vi "Execute New VI From Template.vi"(6 "Mouse Position":T2, 8 "User VI Ref":refnum<vi>, 9 "Menu Item Tag Suffix":string, 10 "Remaining Items":refnum<vi>[](array[refnum]), 11 "Affected Items":cluster{"Any Refnums":refnum<vi>[]}) -> (0 "Fail transaction?":bool)   [LabVIEW 2022 SP3]
doc: "This is the main VI of the \"New VI From Template\" shortcut menu plugin.\n\nNotes from shortcut menu template VI:\n1. This VI has no need for a Close Reference call because GObject refnums do not hold the VI in memory. The User VI Ref will be closed by the caller.\n2. You may enable debugging on this VI to help develop your code. Debugging only has to be disabled on the builder VI, not the execute VI.\n\nPetru Tarabuta, Robusto Systems, September 2022"
uses:
  <vilib>/Utility/miscctls.llb/LVPositionTypeDef.ctl
  Owner Status (enum).ctl
  GUI Objects (cluster).ctl
  Testing Flag (enum).ctl
  Testing Flag (library variable).vi
  <resource>/Framework/Providers/VILibrary/LIBUIP_item_type.ctl
panel:
  out "Application Name":string
  out "VI Of Top-Most Block Diagram":string
  out "This Application Reference":u32
  out "Application Name":string
  out "VI Of Top-Most Block Diagram":string
  out "This Application Reference":u32
  in  "SCL":i32(listbox) caption="Template VIs and CTLs"
  in  "Apply Owner Icon Template?":bool
  out "Error Out":errorcluster
  out "Owner Filename (including extension)":string
  out "User VI Owner Status":T1
  out "Owner Path":path
  out "Iteration":i32
  out "Tab":enum32{"SomeTemplatesFound", "NoTemplatesFound"}(tab)
  in  "Insert into Virtual Folder?":bool
  in  "Create Button":bool
  in  "Destination Location":path caption="Destination Folder"
  in  "Project ComboBox":string(combo) caption="Project"
  in  "New Filename":string
  in  "VI Description":string
  in  "Add To Project?":bool
  in  "Add To Owner?":bool caption="Add to Class 1.lvclass?"
  in  "Open Front Panel?":bool caption="Open Front Panel When Created?"
  out "Virtual Folder Path":string
  out "NoTemplatesFound Message":string
  in  "Front Panel Sizing Tool":bool
  # "Execute VI"
  # "The tool's Application Instance"
  # "The User VI's Application Instance"
  # "The section below is not user-facing. For developer use only."
  # "All controls on this panel except \"Affected Items\" have been locked to prevent accidental edits. Changing the control names or types, other than the elements of the \"Affected Items\" cluster will make the VI unusable as a menu plugin.\n\nSee Context Help for each control for details about its use."
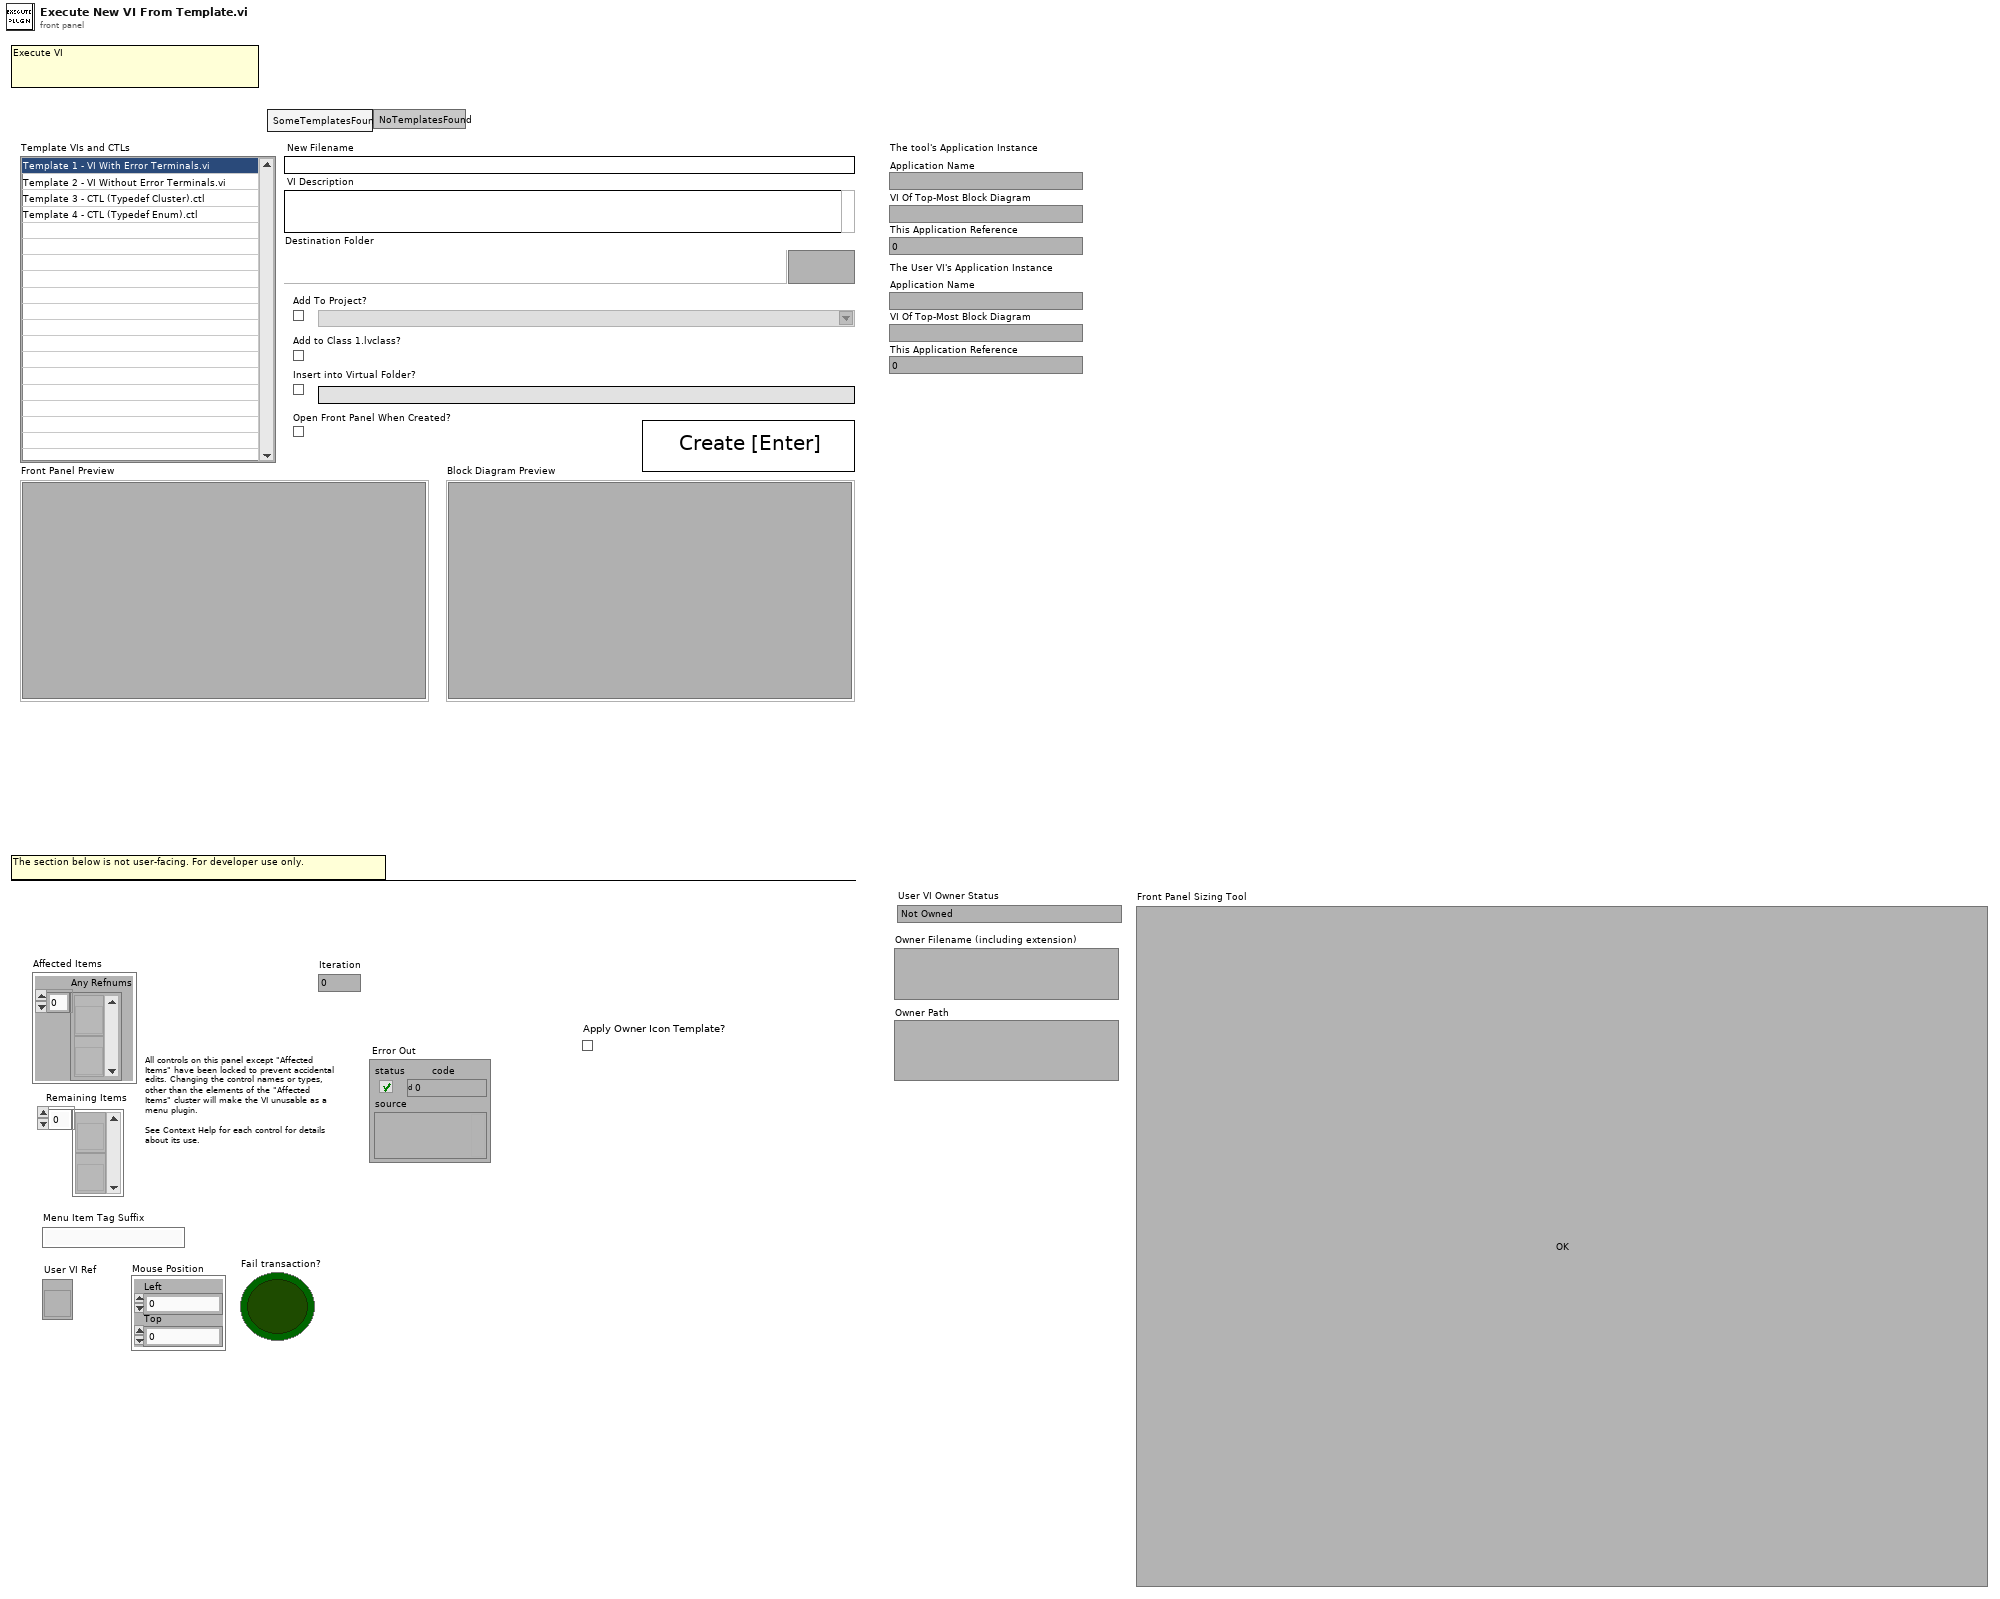
[diagram p1: front panel]
types:
  T1 = typedef "Owner Status (enum).ctl" = enum16{"Not Owned", "Owned by Library (lvlib)", "Owned by Class (lvclass)"}
  T2 = typedef "LVPositionTypeDef.ctl" = cluster{"Left":i32, "Top":i32}
  T3 = typedef "GUI Objects (cluster).ctl" = cluster{"SCL":refnum<vi>, "Add To Owner?":refnum<vi>, "Add To Project?":refnum<vi>, "Open Front Panel?":refnum<vi>, "Destination Folder":refnum<vi>, "Create Button":refnum<vi>, "Project ComboBox":refnum<vi>, "NoTemplatesFound Message":refnum<vi>, "Diagram Preview Subpanel":refnum<vi>, "Insert into Virtual Folder?":refnum<vi>, "Virtual Folder Path":refnum<vi>, "New Filename":refnum<vi>, "VI Description":refnum<vi>}
  T4 = typedef "Testing Flag (enum).ctl" = enum16{"Production", "Testing"}
  T5 = typedef "DFS Output (cluster).ctl" = cluster{"Was File Found?":bool, "Project Item Ref (The VI)":refnum<vi>, "Project Item Ref (Containing Folder)":refnum<vi>, "Folder Path":string, "Was Search Aborted?":bool}
  T6 = typedef "LIBUIP_item_type.ctl" = enum16{"None", "ParentLib", "Property Def Item", "VI", "Non-VI", "Folder", "Library", "Menu", "XI Ability VI", "XI Method VI", "XI Property VI", "Property Folder", "Class Private Data"}
  T7 = enum8{"Enabled", "Disabled", "Disabled and Grayed Out"}
  T8 = enum32{"Invalid", "Standard", "Closed", "Hidden", "Minimized", "Maximized"}
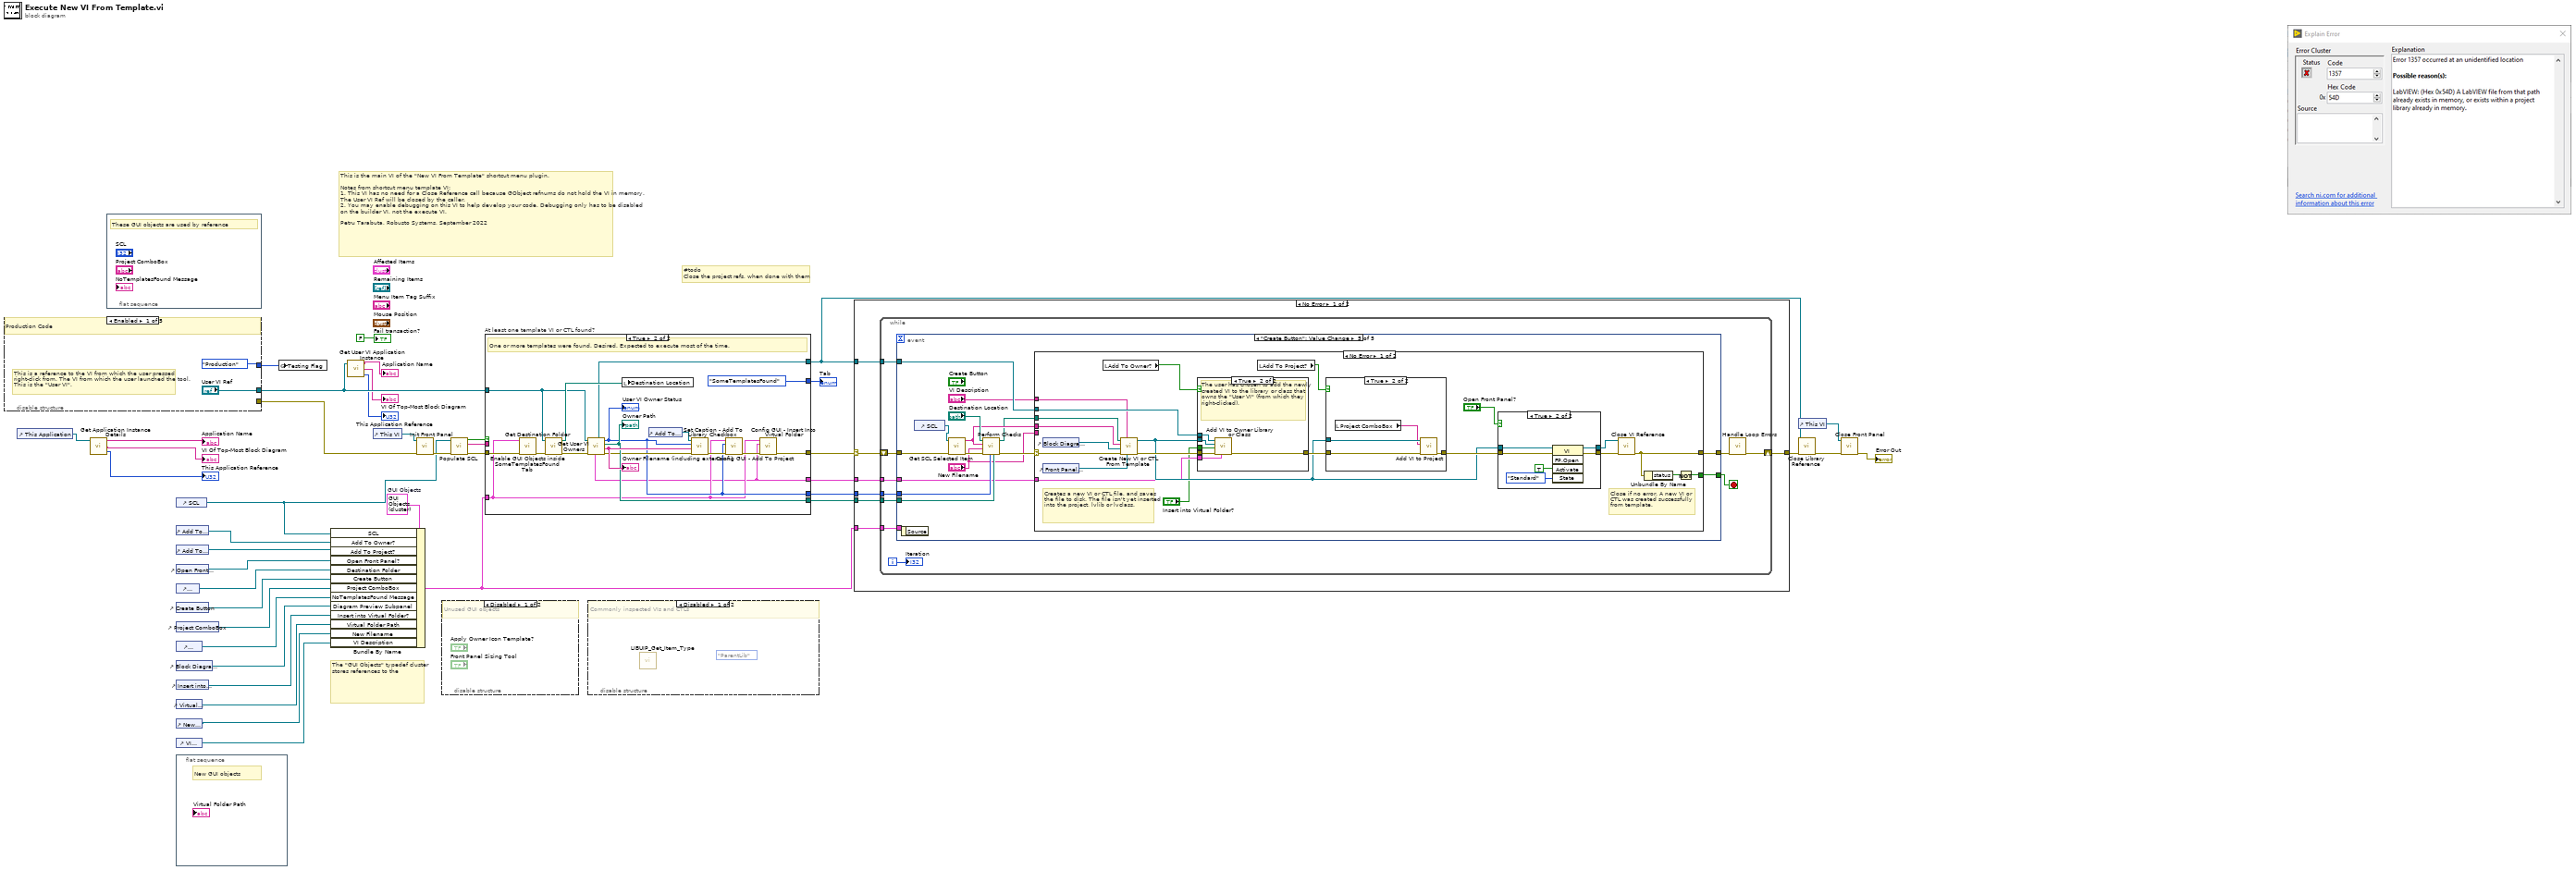
[diagram p0: block diagram]
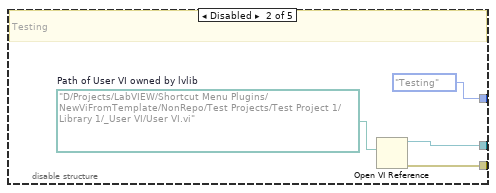
[diagram p3: hidden frame]
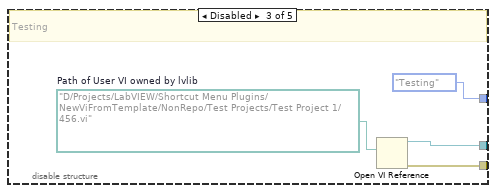
[diagram p4: hidden frame]
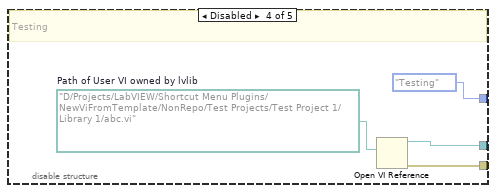
[diagram p5: hidden frame]
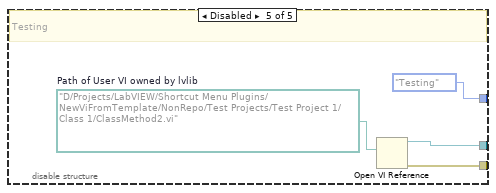
[diagram p6: hidden frame]
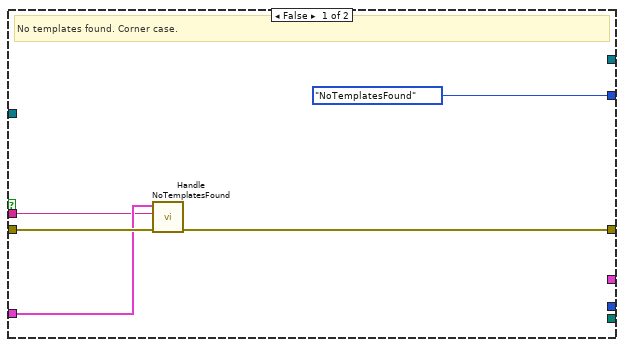
[diagram p7: hidden frame]
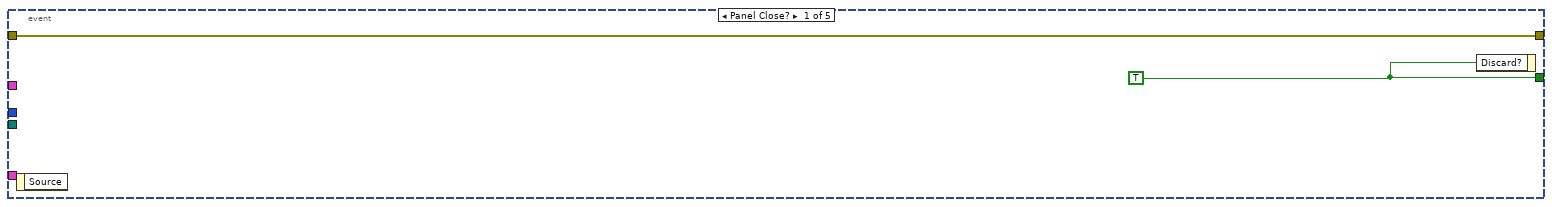
[diagram p9: hidden frame]
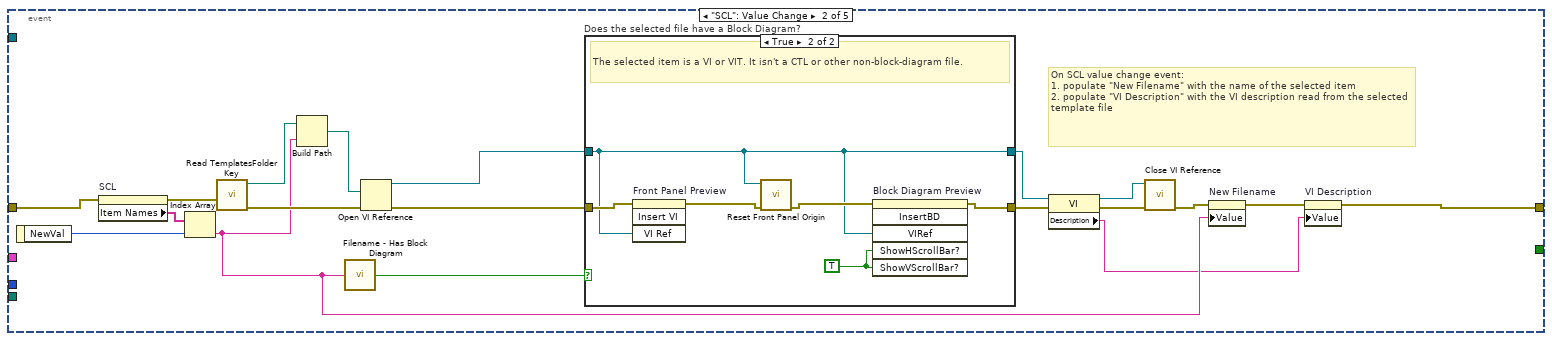
[diagram p10: hidden frame]
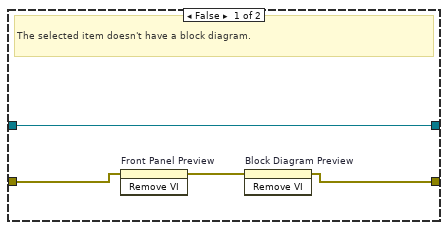
[diagram p11: hidden frame]
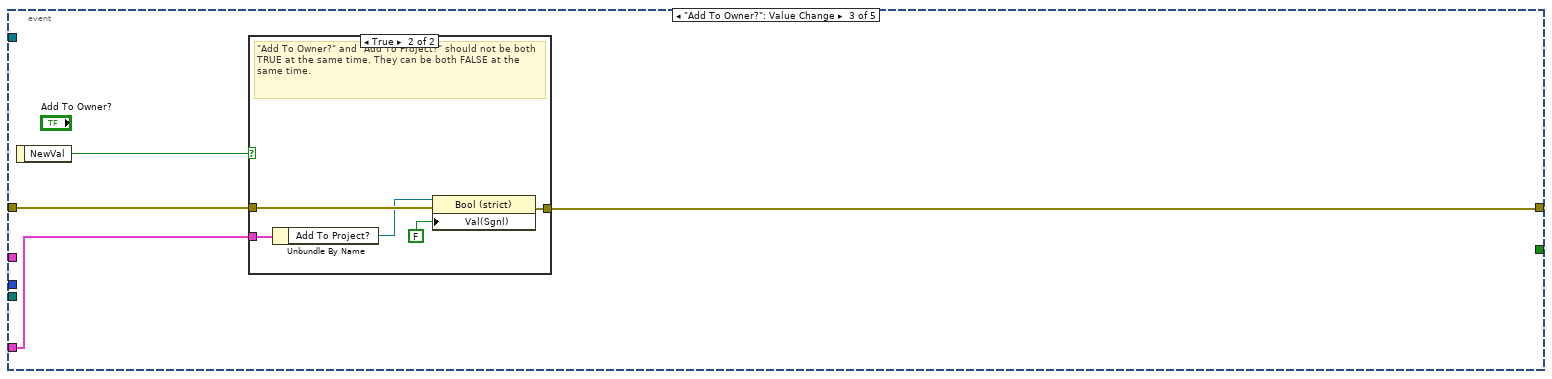
[diagram p12: hidden frame]
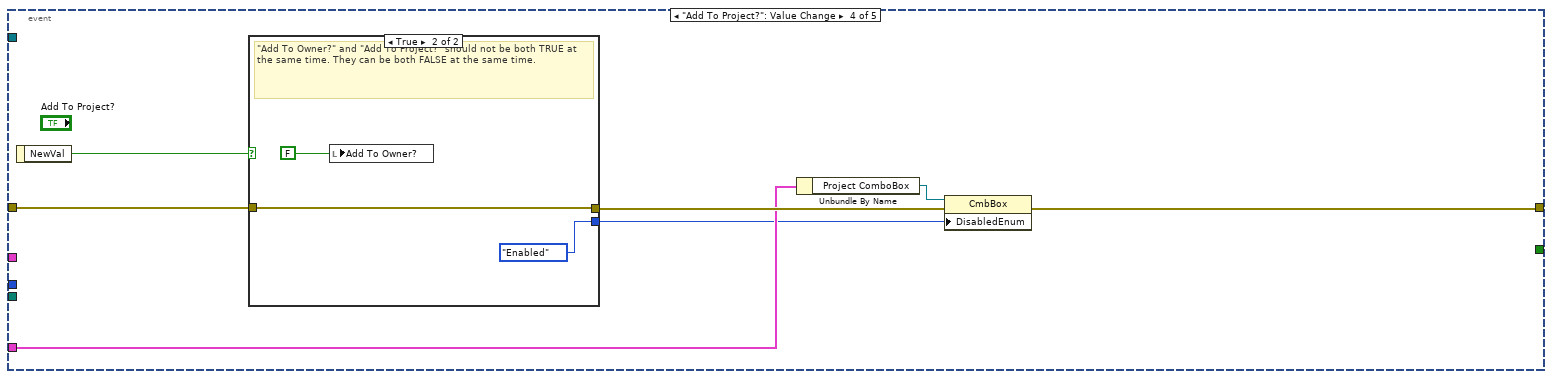
[diagram p14: hidden frame]
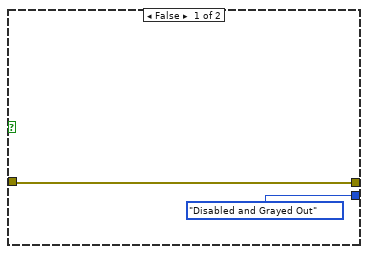
[diagram p15: hidden frame]
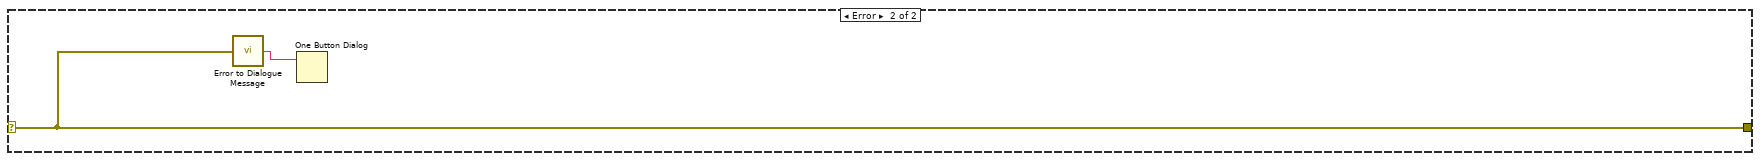
[diagram p20: hidden frame]
diagram:
  w34 = T3 {"SCL"=refnum, "Add To Owner?"=refnum, "Add To Project?"=refnum, "Open Front Panel?"=refnum, "Destination Folder"=refnum, "Create Button"=refnum, "Project ComboBox"=refnum, "NoTemplatesFound Message"=refnum, "Diagram Preview Subpanel"=refnum, "Insert into Virtual Folder?"=refnum, "Virtual Folder Path"=refnum, "New Filename"=refnum, "VI Description"=refnum}  # GUI Objects
  # "#todo\nClose the project refs, when done with them"
  # "The \"GUI Objects\" typedef cluster stores references to the"
  # "This is the main VI of the \"New VI From Template\" shortcut menu plugin.\n\nNotes from shortcut menu template VI:\n1. This VI has no need for a Close Reference call because GObject refnums do not hold the VI in memory. The User VI Ref will be closed by the caller.\n2. You may enable debugging on this VI to help develop your code. Debugging only has to be disabled on the builder VI, not the execute VI.\n\nPetru Tarabuta, Robusto Systems, September 2022"
  n1 = disable-structure shown="Enabled" {
    disable-tunnel: ["User VI Ref" w45 w49 w53 w57] -> w4
    disable-tunnel: [Testing_Flag_(enum)."Production" ("Testing Flag") Testing_Flag_(enum)."Testing" ("Testing Flag") Testing_Flag_(enum)."Testing" ("Testing Flag") Testing_Flag_(enum)."Testing" ("Testing Flag") Testing_Flag_(enum)."Testing" ("Testing Flag")] -> w26
    disable-tunnel: [_ w44 w48 w52 w56] -> w24
    frame Enabled {
      # "This is a reference to the VI from which the user pressed right-click from. The VI from which the user launched the tool. This is the \"User VI\"."
      # "Production Code"
    }
    frame Disabled {
      w46 = path "D:/Projects/LabVIEW/Shortcut Menu Plugins/NewViFromTemplate/NonRepo/Test Projects/Test Project 1/Library 1/_User VI/User VI.vi"  # Path of User VI owned by lvlib
      # "Testing"
      n2 = Open VI Reference(vi path=w46) -> (vi reference=w45:refnum<vi>, error out=w44:errorcluster)  [unwired: 5 in]
    }
    frame Disabled {
      w50 = path "D:/Projects/LabVIEW/Shortcut Menu Plugins/NewViFromTemplate/NonRepo/Test Projects/Test Project 1/456.vi"  # Path of User VI owned by lvlib
      # "Testing"
      n3 = Open VI Reference(vi path=w50) -> (vi reference=w49:refnum<vi>, error out=w48:errorcluster)  [unwired: 5 in]
    }
    frame Disabled {
      w54 = path "D:/Projects/LabVIEW/Shortcut Menu Plugins/NewViFromTemplate/NonRepo/Test Projects/Test Project 1/Library 1/abc.vi"  # Path of User VI owned by lvlib
      # "Testing"
      n4 = Open VI Reference(vi path=w54) -> (vi reference=w53:refnum<vi>, error out=w52:errorcluster)  [unwired: 5 in]
    }
    frame Disabled {
      w58 = path "D:/Projects/LabVIEW/Shortcut Menu Plugins/NewViFromTemplate/NonRepo/Test Projects/Test Project 1/Class 1/ClassMethod2.vi"  # Path of User VI owned by lvlib
      # "Testing"
      n5 = Open VI Reference(vi path=w58) -> (vi reference=w57:refnum<vi>, error out=w56:errorcluster)  [unwired: 5 in]
    }
  }
  n6 = control-ref of="This Application"() -> (w5:refnum<vi>)
  n7 = call "Get Application Instance Details.vi"("Application Instance Ref"=w5) -> ("This Application Reference"=→"This Application Reference":u32, "VI Of Top-Most Block Diagram"=→"VI Of Top-Most Block Diagram":string, "Application Name"=→"Application Name":string)  [unwired: 2 in]
  n8 = flat-sequence {
    frame #0 {
      # "These GUI objects are used by reference"
    }
  }
  n9 = control-ref of="SCL"() -> (w16:refnum<vi>)
  n10 = control-ref of="Add To Owner?"() -> (w33:refnum<vi>)
  n11 = control-ref of="Add To Project?"() -> (w30:refnum<vi>)
  n12 = control-ref of="Open Front Panel?"() -> (w29:refnum<vi>)
  n13 = control-ref of="Destination Location"() -> (w32:refnum<vi>)
  n14 = control-ref of="Create Button"() -> (w31:refnum<vi>)
  n15 = control-ref of="Project ComboBox"() -> (w23:refnum<vi>)
  n16 = control-ref of="NoTemplatesFound Message"() -> (w18:refnum<vi>)
  n17 = control-ref of="Block Diagram Preview"() -> (w17:refnum<vi>)
  n18 = control-ref of="Insert into Virtual Folder?"() -> (w14:refnum<vi>)
  n19 = control-ref of="Virtual Folder Path"() -> (w13:refnum<vi>)
  n20 = control-ref of="New Filename"() -> (w12:refnum<vi>)
  n21 = control-ref of="VI Description"() -> (w11:refnum<vi>)
  n22 = flat-sequence {
    frame #0 {
      # "New GUI objects"
    }
  }
  n23 = global write "Testing Flag (library variable).vi" "Testing Flag"(w26) -> ()
  n24 = Bundle By Name(cluster=w34, "SCL"=w16, "Add To Owner?"=w33, "Add To Project?"=w30, "Open Front Panel?"=w29, "Destination Folder"=w32, "Create Button"=w31, "Project ComboBox"=w23, "NoTemplatesFound Message"=w18, "Diagram Preview Subpanel"=w17, "Insert into Virtual Folder?"=w14, "Virtual Folder Path"=w13, "New Filename"=w12, "VI Description"=w11) -> (w21:T3)
  n25 = call "Get User VI Application Instance.vi"("User VI Ref"=w4) -> ("This Application Reference"=→"This Application Reference":u32, "VI Of Top-Most Block Diagram"=→"VI Of Top-Most Block Diagram":string, "Application Name"=→"Application Name":string)  [unwired: 2 in]
  n26 = control-ref of="This VI"() -> (w40:refnum<vi>)
  n27 = call "Init Front Panel.vi"("error in"=w24, "VI Reference"=w40) -> ("error out"=w39:errorcluster)  [unwired: 9 in]
  n28 = disable-structure shown="Disabled" {
    frame Disabled {
      # "Unused GUI objects"
    }
    frame Enabled {
    }
  }
  n29 = call "Populate SCL.vi"("error in"=w39, "SCL"=w16) -> ("error out"=w28:errorcluster, "No Templates Found Message"=w15:string, "At least one template file found?"=w20:bool)  [unwired: 7 in]
  n30 = case "At least one template VI or CTL found?" shown="True" w20 {
    tunnel: [_ w76] -> w35
    tunnel: w4 -> [_ w75]
    tunnel: w28 -> [w64 w73]
    tunnel: [_ w68] -> w27
    tunnel: [_ w72] -> w10
    tunnel: [w62 w67] -> w22
    tunnel: w21 -> [w61 w66]
    tunnel: [enum32{"SomeTemplatesFound", "NoTemplatesFound"}."NoTemplatesFound" ("Tab") enum32{"SomeTemplatesFound", "NoTemplatesFound"}."SomeTemplatesFound" ("Tab")] -> w19
    tunnel: w15 -> [w60 _]
    tunnel: [_ w65] -> w9
    frame False {
      # "No templates found. Corner case."
      n31 = call "Handle NoTemplatesFound.vi"("error in"=w64, "No Templates Found Message"=w60, "GUI Objects"=w61) -> ("error out"=w62:errorcluster)  [unwired: 8 in]
    }
    frame True {
      # "One or more templates were found. Desired. Expected to execute most of the time."
      n32 = call "Enable GUI Objects inside SomeTemplatesFound Tab.vi"("error in"=w73, "GUI Objects"=w66) -> ("error out"=w69:errorcluster)  [unwired: 9 in]
      n33 = call "Get Destination Folder.vi"("error in"=w69, "User VI Ref"=w75) -> ("error out"=w81:errorcluster, "Destination Folder"=w77:path)  [unwired: 8 in]
      n34 = call "Get User VI Owners.vi"("error in"=w81, "User VI Ref"=w75) -> ("error out"=w74:errorcluster, "Owner Filename (inc file extension)"=w78:string, "Owner Path"=w76:path, "User VI Owner Status"=w68:T1, "Owner Reference"=w72:refnum<vi>, "Virtual Folder Search Results"=w65:T5)  [unwired: 3 in, 1 out]
      "Owner Path" <- w76
      "User VI Owner Status" <- w68
      "Owner Filename (including extension)" <- w78
      n35 = local write "Destination Location"(w77) -> ()
      n36 = control-ref of="Add To Owner?"() -> (w79:refnum<vi>)
      n37 = call "Set Caption - Add To Library Checkbox.vi"("error in"=w74, "Owner Filename (including extension)"=w78, "User VI Owner Status"=w68, "Add To Owner"=w79) -> ("error out"=w80:errorcluster)  [unwired: 7 in]
      n38 = call "Config GUI - Add To Project.vi"("error in"=w80, "User VI Owner Status"=w68, "GUI Objects"=w66) -> ("error out"=w71:errorcluster)  [unwired: 7 in, 1 out]
      n39 = call "Config GUI - Insert Into Virtual Folder.vi"("error in"=w71, "Virtual Folder Search Results"=w65, "GUI Objects"=w66) -> ("error out"=w67:errorcluster)  [unwired: 8 in]
    }
  }
  "Tab" <- w19
  n40 = disable-structure shown="Disabled" {
    frame Disabled {
      (unwired) LIBUIP_item_type."ParentLib" ("Type")
      # "Commonly inspected VIs and CTLs"
      n41 = call <resource>:"LIBUIP_Get_Item_Type.vi"() -> ()  [unwired: 2 in, 10 out]
    }
    frame Enabled {
    }
  }
  n42 = case shown="No Error" w22 {
    selector: w22 -> [w88 w210]
    tunnel: [w87 w210] -> w38
    tunnel: w27 -> [w86 _]
    tunnel: w35 -> [w85 _]
    tunnel: w21 -> [w84 _]
    tunnel: w10 -> [w83 _]
    tunnel: w9 -> [w82 _]
    frame No Error {
      n43 = while {
        shift-right: [w92] -> w87
        shift-left: w88 -> [w98]
        tunnel: w86 -> [w95]
        tunnel: w85 -> [w94]
        tunnel: w84 -> [w91]
        tunnel: w83 -> [w90]
        tunnel: w82 -> [w89]
        i -> [w97]
        stop <- w96 stop-if-true
        n44 = event shown="[4] \"Create Button\": Value Change" {
          selector: _ -> [_ _ _ _ _]
          dyn-events: _ -> [_ _ _ _ _]
          timeout: _ -> [_ _ _ _ _]
          tunnel: w98 -> [w99 w119 w132 w145 w165]
          tunnel: [w100 _ _ _ w157] -> w96
          tunnel: [w99 w102 w131 w143 w166] -> w93
          tunnel: w95 -> [_ _ _ _ w162]
          tunnel: w94 -> [_ _ _ _ w161]
          tunnel: w91 -> [_ _ w130 w142 _]
          tunnel: w90 -> [_ _ _ _ w158]
          tunnel: w89 -> [_ _ _ _ w152]
          event Panel Close? {
            w100 = TRUE
            n45 = event-data() -> ()  [unwired: 1 in, 1 out]
            n46 = event-data("Discard?"=w100) -> ()  [unwired: 1 in, 1 out]
          }
          event "SCL": Value Change {
            # "On SCL value change event: \n1. populate \"New Filename\" with the name of the selected item\n2. populate \"VI Description\" with the VI description read from the selected template file"
            n47 = event-data() -> ("NewVal"=w117:i32)  [unwired: 1 in]
            n48 = property on="SCL" class="LstBox (strict)"(error in=w119) -> (error out=w116:errorcluster, "Item Names"=w118:string[])  [unwired: 1 in, 1 out]
            n49 = Index Array(array=w118, index=w117) -> (element=w107:string)
            n50 = call "Read TemplatesFolder Key.vi"("Error In"=w116) -> ("Error Out"=w113:errorcluster, "Templates Folder Path"=w115:path)  [unwired: 9 in]
            n51 = Build Path(base path=w115, name or relative path=w107) -> (appended path=w114:path)
            n52 = call "Filename - Has Block Diagram.vi"("Filename (including file extension)"=w107) -> ("Has Block Diagram?"=w111:bool)
            n53 = Open VI Reference(vi path=w114, error in (no error)=w113) -> (vi reference=w112:refnum<vi>, error out=w108:errorcluster)  [unwired: 4 in]
            n54 = case "Does the selected file have a Block Diagram?" shown="True" w111 {
              tunnel: [w123 w128] -> w110
              tunnel: w112 -> [w122 w124]
              tunnel: [w122 w124] -> w105
              tunnel: w108 -> [w120 w127]
              frame False {
                # "The selected item doesn't have a block diagram."
                n55 = invoke on="Front Panel Preview" class="SubPnl" method="Remove VI"(error in=w120) -> (error out=w121:errorcluster)  [unwired: 2 in, 2 out]
                n56 = invoke on="Block Diagram Preview" class="SubPnl" method="Remove VI"(error in=w121) -> (error out=w123:errorcluster)  [unwired: 2 in, 2 out]
              }
              frame True {
                w129 = TRUE ("ShowHScrollBar")
                # "The selected item is a VI or VIT. It isn't a CTL or other non-block-diagram file."
                n57 = invoke on="Front Panel Preview" class="SubPnl" method="Insert VI"(error in=w127, "VI Ref"=w124) -> (error out=w126:errorcluster)  [unwired: 2 in, 3 out]
                n58 = call "Reset Front Panel Origin.vi"("Error In"=w126, "VI Reference"=w124) -> ("Error Out"=w125:errorcluster)  [unwired: 9 in]
                n59 = invoke on="Block Diagram Preview" class="SubPnl" method="InsertBD"(error in=w125, "VIRef"=w124, "ShowHScrollBar?"=w129, "ShowVScrollBar?"=w129) -> (error out=w128:errorcluster)  [unwired: 2 in, 5 out]
              }
            }
            n60 = property class="VI"(reference=w105, error in=w110) -> (reference out=w104:refnum<vi>, error out=w106:errorcluster, "Description"=w101:string)
            n61 = call "Close VI Reference.vi"("error in"=w106, "VI Reference"=w104) -> ("error out"=w109:errorcluster)  [unwired: 9 in]
            n62 = property on="New Filename" class="Str"(error in=w109, "Value"=w107) -> (error out=w103:errorcluster)  [unwired: 1 in, 1 out]
            n63 = property on="VI Description" class="Str"(error in=w103, "Value"=w101) -> (error out=w102:errorcluster)  [unwired: 1 in, 1 out]
          }
          event "Add To Owner?": Value Change {
            n64 = event-data() -> ("NewVal"=w133:bool)  [unwired: 1 in]
            n65 = case shown="True" w133 {
              tunnel: w132 -> [w134 w139]
              tunnel: [w134 w138] -> w131
              tunnel: w130 -> [_ w137]
              frame False {
              }
              frame True {
                # "\"Add To Owner?\" and \"Add To Project?\" should not be both TRUE at the same time. They can be both FALSE at the same time."
                n66 = Unbundle By Name(w137) -> ("Add To Project?"=w136:refnum<vi>)
                n67 = property class="Bool (strict)"(reference=w136, error in=w139, "Val(Sgnl)"=FALSE ("Value (Signaling)")) -> (error out=w138:errorcluster)  [unwired: 1 out]
              }
            }
          }
          event "Add To Project?": Value Change {
            n68 = event-data() -> ("NewVal"=w146:bool)  [unwired: 1 in]
            n69 = case shown="True" w146 {
              tunnel: w145 -> [w148 w150]
              tunnel: [w148 w150] -> w144
              tunnel: [T7."Disabled and Grayed Out" ("Disabled") T7."Enabled" ("Disabled")] -> w140
              frame False {
              }
              frame True {
                # "\"Add To Owner?\" and \"Add To Project?\" should not be both TRUE at the same time. They can be both FALSE at the same time."
                n70 = local write "Add To Owner?"(FALSE ("Add To Project?")) -> ()
              }
            }
            n71 = Unbundle By Name(w142) -> ("Project ComboBox"=w141:refnum<vi>)
            n72 = property class="CmbBox"(reference=w141, error in=w144, "DisabledEnum"=w140) -> (error out=w143:errorcluster)  [unwired: 1 out]
          }
          event "Create Button": Value Change {
            n73 = event-data() -> ()  [unwired: 1 in, 1 out]
            n74 = control-ref of="SCL"() -> (w156:refnum<vi>)
            n75 = call "Get SCL Selected Item.vi"("error in"=w165, "SCL"=w156) -> ("error out"=w164:errorcluster, "Selected Item (String)"=w159:string)  [unwired: 7 in, 1 out]
            n76 = call "Perform Checks.vi"("Owner Path (if applicable)"=w161, "User VI Owner Status"=w162, "error in"=w164, "New Filename"="New Filename", "Selected Template VI or CTL name (including file extension)"=w159, "Destination Folder"="Destination Location") -> ("error out"=w163:errorcluster, "Filepath of VI or CTL to be created"=w153:path)  [unwired: 3 in, 1 out]
            n77 = case shown="No Error" w163 {
              selector: w163 -> [w187 w208]
              tunnel: [w176 w208] -> w166
              tunnel: w159 -> [w186 _]
              tunnel: w158 -> [w183 _]
              tunnel: [w174 _] -> w157
              tunnel: "New Filename" -> [_ _]
              tunnel: "VI Description" -> [w171 _]
              tunnel: w153 -> [w170 _]
              tunnel: w152 -> [w168 _]
              frame No Error {
                # "Close if no error. A new VI or CTL was created successfully from template."
                # "Creates a new VI or CTL file, and saves the file to disk. The file isn't yet inserted into the project, lvlib or lvclass."
                n78 = control-ref of="Block Diagram Preview"() -> (w173:refnum<vi>)
                n79 = control-ref of="Front Panel Preview"() -> (w172:refnum<vi>)
                n80 = local read "Add To Owner?"() -> (w185:bool)
                n81 = call "Create New VI or CTL From Template.vi"("Front Panel Preview"=w172, "VI Description"=w171, "error in"=w187, "Block Diagram Preview (Subpanel Ref)"=w173, "Selected Template VI or CTL name (including file extension)"=w186, "Filepath of VI or CTL to be created"=w170) -> ("error out"=w184:errorcluster, "Reference of newly created VI"=w177:refnum<vi>)  [unwired: 4 in]
                n82 = case shown="True" w185 {
                  tunnel: [w193 w199] -> w180
                  tunnel: w184 -> [w193 w198]
                  tunnel: w177 -> [_ w197]
                  tunnel: w183 -> [_ w196]
                  tunnel: w168 -> [_ w195]
                  tunnel: "Insert into Virtual Folder?" -> [_ w194]
                  frame False {
                  }
                  frame True {
                    # "The user has chosen to add the newly created VI to the library or class that owns the \"User VI\" (from which they right-clicked)."
                    n83 = call "Add VI to Owner Library or Class.vi"("Virtual Folder Search Results"=w195, "error in"=w198, "Insert into Virtual Folder?"=w194, "Reference of newly created VI"=w197, "Owner Reference (Library or Class)"=w196) -> ("error out"=w199:errorcluster)  [unwired: 6 in]
                  }
                }
                n84 = local read "Add To Project?"() -> (w178:bool)
                n85 = case shown="True" w178 {
                  tunnel: [w188 w192] -> w179
                  tunnel: w180 -> [w188 w191]
                  tunnel: w177 -> [_ w190]
                  frame False {
                  }
                  frame True {
                    n86 = local read "Project ComboBox"() -> (w189:string)
                    n87 = call "Add VI to Project.vi"("error in"=w191, "Project Name"=w189, "Reference of newly created VI or CTL"=w190) -> ("error out"=w192:errorcluster)  [unwired: 8 in]
                  }
                }
                n88 = case shown="True" "Open Front Panel?" {
                  tunnel: w179 -> [w201 w207]
                  tunnel: [w201 w206] -> w182
                  tunnel: w177 -> [w200 w205]
                  tunnel: [w200 w202] -> w181
                  frame False {
                  }
                  frame True {
                    n89 = invoke class="VI" method="FP.Open"(reference=w205, error in=w207, "Activate"=TRUE ("Activate?"), "State"=T8."Standard") -> (reference out=w202:refnum<vi>, error out=w206:errorcluster)  [unwired: 1 in, 3 out]
                  }
                }
                n90 = call "Close VI Reference.vi"("error in"=w182, "VI Reference"=w181) -> ("error out"=w176:errorcluster)  [unwired: 9 in]
                n91 = Unbundle By Name(w176) -> ("status"=w175:bool)
                n92 = Not(x=w175) -> (.not. x?=w174:bool)
              }
              frame Error {
              }
            }
          }
        }
        n93 = call "Handle Loop Errors.vi"("error in"=w93) -> ("error out"=w92:errorcluster)  [unwired: 10 in]
        "Iteration" <- w97
      }
    }
    frame Error {
      n94 = call "Error to Dialogue Message.vi"("error in"=w210) -> ("Dialogue Message"=w209:string)
      n95 = One Button Dialog(message=w209) -> ()  [unwired: 1 in, 1 out]
    }
  }
  n96 = control-ref of="This VI"() -> (w37:refnum<vi>)
  n97 = call "Close Library Reference.vi"("error in"=w38, "Library Owner Reference"=w10) -> ("error out"=w25:errorcluster)  [unwired: 9 in]
  n98 = call "Close Front Panel.vi"("error in"=w25, "VI Reference"=w37) -> ("error out"=→"Error Out":errorcluster)  [unwired: 9 in]
  "Fail transaction?" <- FALSE ("Fail transaction?")
